vi "Intensity Graph to XY Graph (Horizontal) (by val).vi"(8 "error in (no error)":errorcluster, 10 "2D Data":dbl[][](array[numeric]), 11 "graph_utilities in":refnum<class "graph_utilities.lvclass">) -> (0 "error out":errorcluster, 2 "XY-data":cluster{"X-array":dbl[], "Y-array":dbl[]}[](array[cluster]), 3 "graph_utilities out":refnum<class "graph_utilities.lvclass">)   [LabVIEW 2019, in "graph_utilities.lvclass"]
doc: "Converts an Intensity Graph into a sequence of plots on a XY Graph.\n\nThe x-axis of the XY Graph will be equal to the x-axis of the Intensity Graph."
uses:
  graph_utilities.lvclass
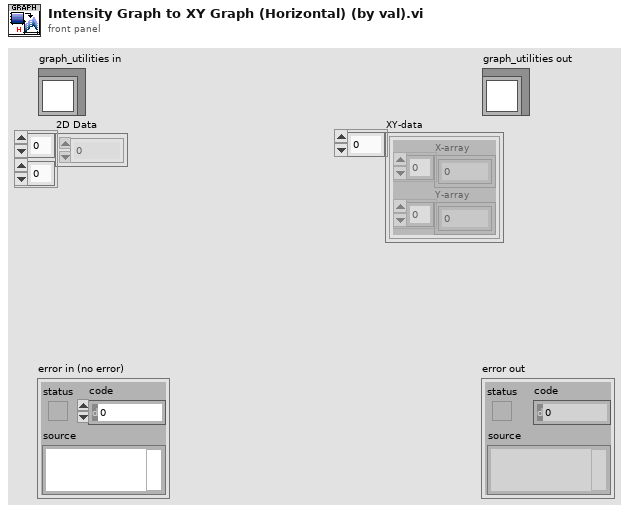
[diagram p1: front panel]
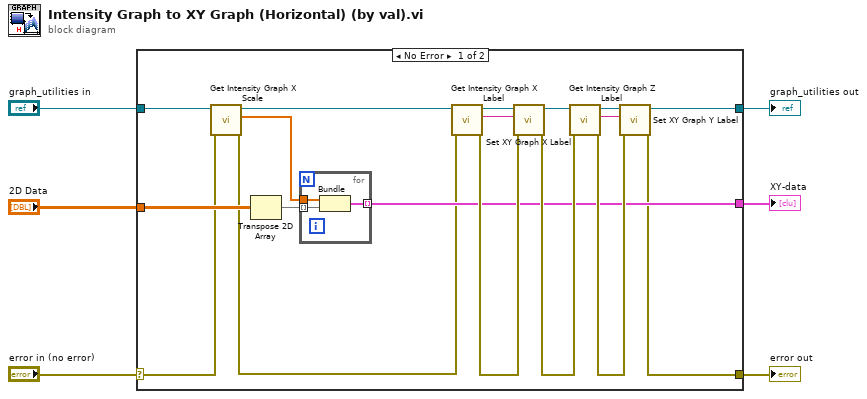
[diagram p0: block diagram]
diagram:
  n1 = case shown="No Error" "error in (no error)" {
    selector: "error in (no error)" -> [w8 w29]
    tunnel: [w9 w29] -> w5
    tunnel: [w15 w28] -> w3
    tunnel: "graph_utilities in" -> [w12 w28]
    tunnel: "2D Data" -> [w13 _]
    tunnel: [w11 _] -> w1
    frame No Error {
      n2 = call "Get Intensity Graph X Scale.vi"("error in (no error)"=w8, "graph_utilities in"=w12) -> ("error out"=w7:errorcluster, "X Scale"=w10:dbl[], "graph_utilities out"=w24:refnum<class "graph_utilities.lvclass">)  [unwired: 6 in, 1 out]
      n3 = Transpose 2D Array(2D array=w13) -> (transposed array=w14:dbl[][])
      n4 = for {
        tunnel: w14 -> [w26] mode=indexing
        tunnel: w10 -> [w27]
        tunnel: [w25] -> w11 mode=indexing
        n5 = Bundle("X Scale"=w27, w26) -> (w25:cluster{"X Scale":dbl[], dbl[]})  [unwired: 1 in]
      }
      n6 = call "Get Intensity Graph X Label.vi"("error in (no error)"=w7, "graph_utilities in"=w24) -> ("error out"=w17:errorcluster, "X Label"=w23:string, "graph_utilities out"=w18:refnum<class "graph_utilities.lvclass">)  [unwired: 7 in]
      n7 = call "Set XY Graph X Label.vi"("error in (no error)"=w17, "X Label"=w23, "graph_utilities in"=w18) -> ("error out"=w19:errorcluster, "graph_utilities out"=w20:refnum<class "graph_utilities.lvclass">)  [unwired: 7 in]
      n8 = call "Get Intensity Graph Z Label.vi"("error in (no error)"=w19, "graph_utilities in"=w20) -> ("error out"=w16:errorcluster, "Z Label"=w22:string, "graph_utilities out"=w21:refnum<class "graph_utilities.lvclass">)  [unwired: 7 in]
      n9 = call "Set XY Graph Y Label.vi"("error in (no error)"=w16, "Y Label"=w22, "graph_utilities in"=w21) -> ("error out"=w9:errorcluster, "graph_utilities out"=w15:refnum<class "graph_utilities.lvclass">)  [unwired: 7 in]
    }
    frame Error {
    }
  }
  "error out" <- w5
  "graph_utilities out" <- w3
  "XY-data" <- w1
